vi "StandaloneManualValveControl.vi"() -> ()   [LabVIEW 2018]
uses:
  <vilib>/MakerHub/LINX/Public/Peripherals/Digital/Digital Write N Chans.vi
  <vilib>/MakerHub/LINX/Private/Local IO/LinxDigitalWrite.vi
  <vilib>/MakerHub/LINX/Public/Utilities/Check Channel.vi
  <vilib>/MakerHub/LINX/Public/Utilities/Open Serial.vi
  <vilib>/MakerHub/LINX/Private/Utilties/Generate Error.vi
  <vilib>/MakerHub/LINX/LMH-LINX.lvlib
panel:
  out "Error Out":errorcluster
  out "Device Name":string
  in  "error in (no error)":errorcluster
  in  "VISA resource name":refnum<visa-resource-name>
  in  "Manually controlled Valves":u8[](array[numeric])
  out "Open?":bool
  in  "Manual Open":bool
  in  "stop":bool
  # "ALWAYS TERMINATE THE\nPROGRAM WITH THIS STOP BUTTON!"
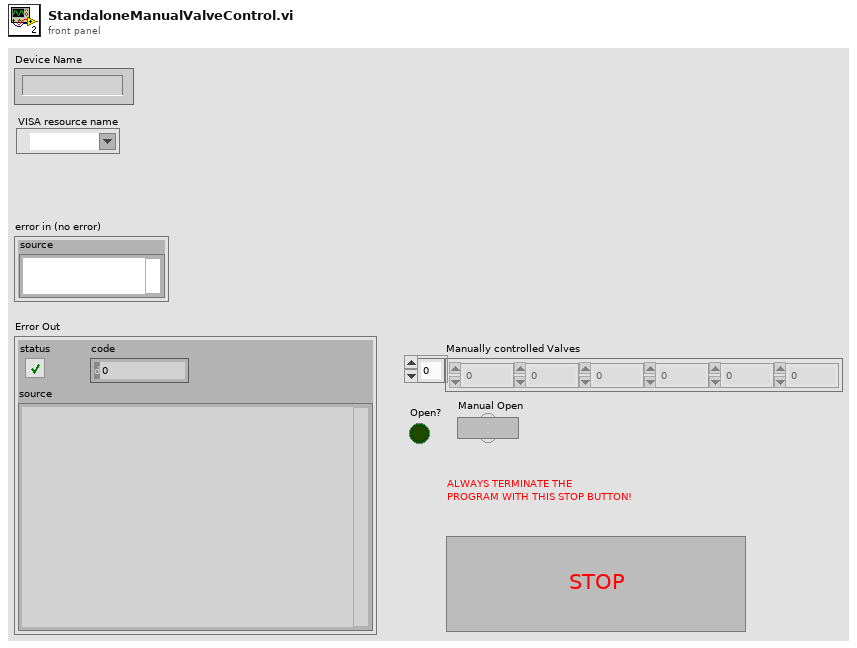
[diagram p1: front panel]
types:
  T1 = typedef "LMH-LINX.lvlib/LINX Ref.ctl" = cluster{"IO":T2, "Interface":T3, "LINX Device Config":T4}
  T2 = typedef "LMH-LINX.lvlib/Platform.ctl" = enum16{"Remote", "Local"}
  T3 = typedef "LMH-LINX.lvlib/Interface.ctl" = enum16{"Serial", "TCP"}
  T4 = typedef "LMH-LINX.lvlib/Device.lvlib/LINX Device Config.ctl" = cluster{"Interface":T3, "COM Port":refnum<visa-resource-name>, "TCP Configuration":T5, "Device Family":u8, "Device ID":u8, "Device Name":string, "TCP Ref":refnum<k5>, "Channels":T6}
  T5 = typedef "LMH-LINX.lvlib/Device.lvlib/TCP Config.ctl" = cluster{"IP Address":string, "Port":u16}
  T6 = typedef "LMH-LINX.lvlib/Channels.ctl" = cluster{"DI":u8[], "DO":u8[], "AI":u8[], "AO":u8[], "PWM":u8[], "QE":u8[], "UART":u8[], "I2C 2":u8[], "SPI":u8[], "CAN":u8[], "Servo":u8[], "AI Ref (V)":dbl, "AI Resolution (Bits)":u8, "AO Ref (V)":dbl, "AO Resolution (Bits)":u8}
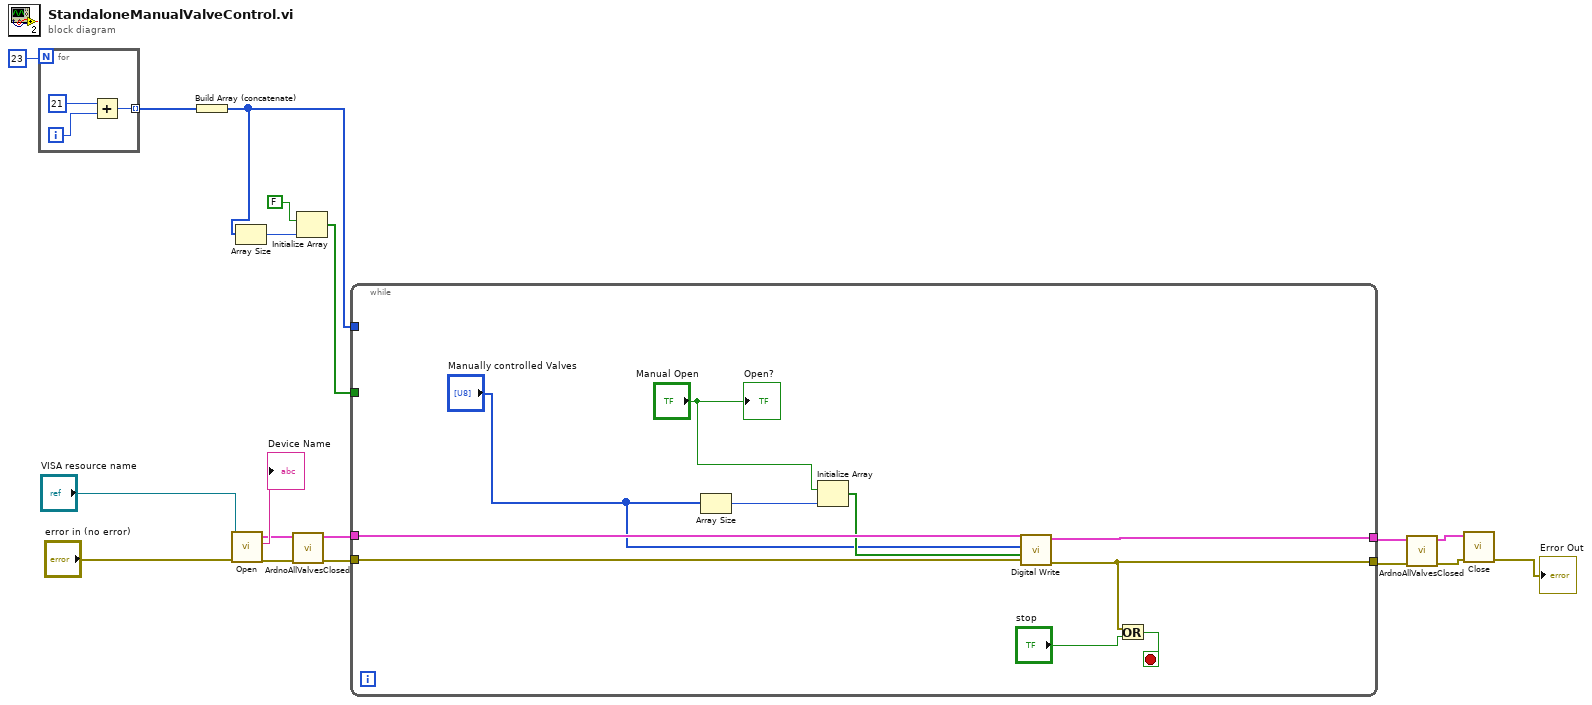
[diagram p0: block diagram]
diagram:
  n1 = for {
    N: 23 -> [_]
    tunnel: [w19] -> w13 mode=indexing
    i -> [w21]
    n2 = Add(x=21, y=w21) -> (x+y=w19:i32)
  }
  n3 = Build Array (concatenate)(w13) -> (w12:i32[])
  n4 = call-poly <vilib>:"Open.vi"("Error In"="error in (no error)", "Serial Port"="VISA resource name") -> ("Error Out"=w1:errorcluster, "Device Name"=→"Device Name":string, "LINX Resource"=w2:T1)  [unwired: 7 in]
  n5 = Array Size(array=w12) -> (size(s)=w11:i32)
  n6 = call "ArdnoAllValvesClosed.vi"("error in (no error)"=w1, "LINX Resource"=w2) -> ("error out"=w3:errorcluster, "LINX Resource out"=w4:T1)  [unwired: 8 in]
  n7 = Initialize Array(FALSE, w11) -> (w9:bool[])
  n8 = while {
    tunnel: w4 -> [w31]
    tunnel: [w30] -> w5
    tunnel: w3 -> [w29]
    tunnel: [w26] -> w6
    tunnel: w12 -> [_]
    tunnel: w9 -> [_]
    stop <- w27 stop-if-true
    n9 = Array Size(array="Manually controlled Valves") -> (size(s)=w25:i32)
    n10 = Initialize Array("Manual Open", w25) -> (w24:bool[])
    n11 = call-poly <vilib>:"Digital Write.vi"("Error In"=w29, "Values"=w24, "DO Channels"="Manually controlled Valves", "LINX Resource"=w31) -> ("Error Out"=w26:errorcluster, "LINX Resource"=w30:T1)  [unwired: 6 in]
    n12 = Or(x=w26, y="stop") -> (x .or. y?=w27:bool)
    "Open?" <- "Manual Open"
  }
  n13 = call "ArdnoAllValvesClosed.vi"("error in (no error)"=w6, "LINX Resource"=w5) -> ("error out"=w7:errorcluster, "LINX Resource out"=w8:T1)  [unwired: 8 in]
  n14 = call <vilib>:"Close.vi"("Error In"=w7, "LINX Resource"=w8) -> ("Error Out"=→"Error Out":errorcluster)  [unwired: 9 in]
